vi "move.vi"   [LabVIEW 2015]
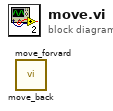
[diagram p0: block diagram]
diagram:
  n1 = call "move_back.vi"() -> ()  [unwired: 1 in, 1 out]
  n2 = call "move_forvard.vi"() -> ()  [unwired: 1 in, 1 out]
